vi "Main.vi"() -> ()   [LabVIEW 2023]
uses:
  CONTROLS/states.ctl
panel:
  in  "stop":bool
  out "Enum":T1
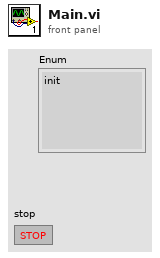
[diagram p1: front panel]
types:
  T1 = typedef "states.ctl" = enum16{"init", "read", "write", "kundeneingabe", "betonauswahl", "bezahlprozess", "rechnung", "zutaten mit gerichtmessung", "stop", ""}
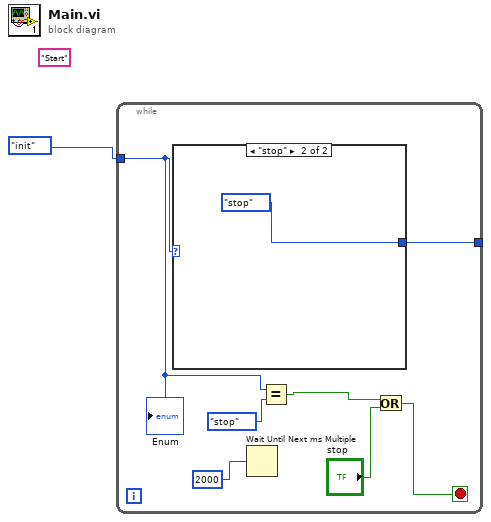
[diagram p0: block diagram]
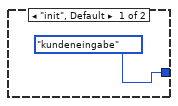
[diagram p2: hidden frame]
diagram:
  (unwired) "Start"
  n1 = while {
    tunnel: states."init" -> [w7]
    tunnel: [w8] -> _
    stop <- w3 stop-if-true
    n2 = case shown="\"stop\"" w7 {
      tunnel: [states."kundeneingabe" states."stop"] -> w8
      frame "init", Default {
      }
      frame "stop" {
      }
    }
    n3 = Wait Until Next ms Multiple(millisecond multiple=2000) -> ()  [unwired: 1 out]
    n4 = Equal?(x=w7, y=states."stop") -> (x = y?=w5:bool)
    n5 = Or(x=w5, y="stop") -> (x .or. y?=w3:bool)
    "Enum" <- w7
  }
